vi "Drift_from_ims.vi"(4 "Filename_2":path, 5 "Python Directory Path":path=path "", 6 "Image Channel":string, 7 "Filename_1":path) -> (0 "Error":sgl, 1 "Shift_z (m/s)":sgl, 2 "Shift_x (m/s)":sgl, 3 "Shift_y (m/s)":sgl)   [LabVIEW 2025]
panel:
  out "result string":string
  out "Shift_z (m)":sgl
  out "standard error":string
  out "Shift_x (m)":sgl
  out "Shift_y (m)":sgl
  out "Time Between Scans":sgl
  out "standard output":string
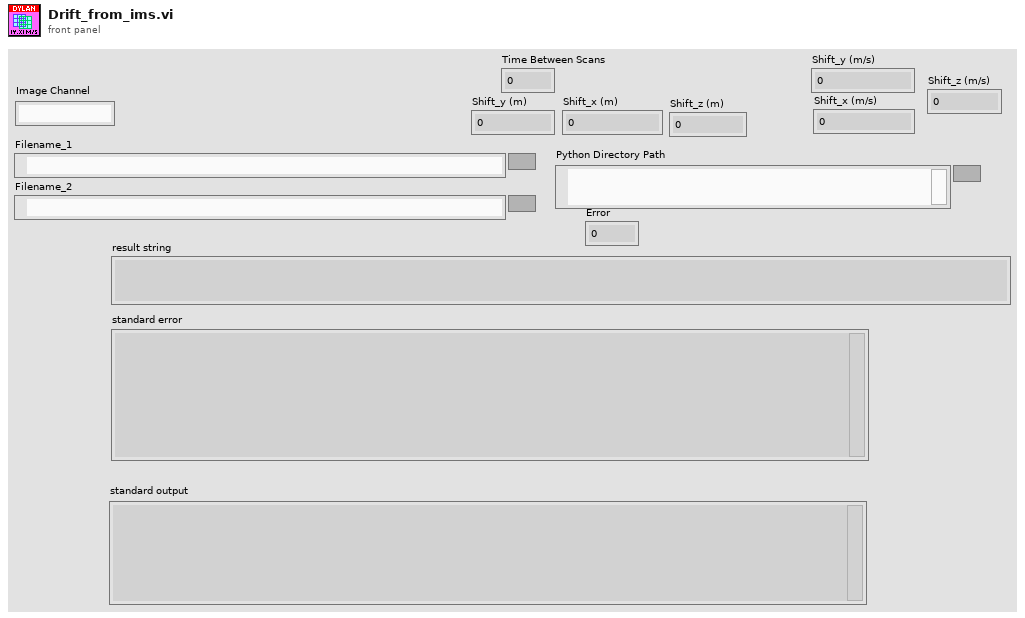
[diagram p1: front panel]
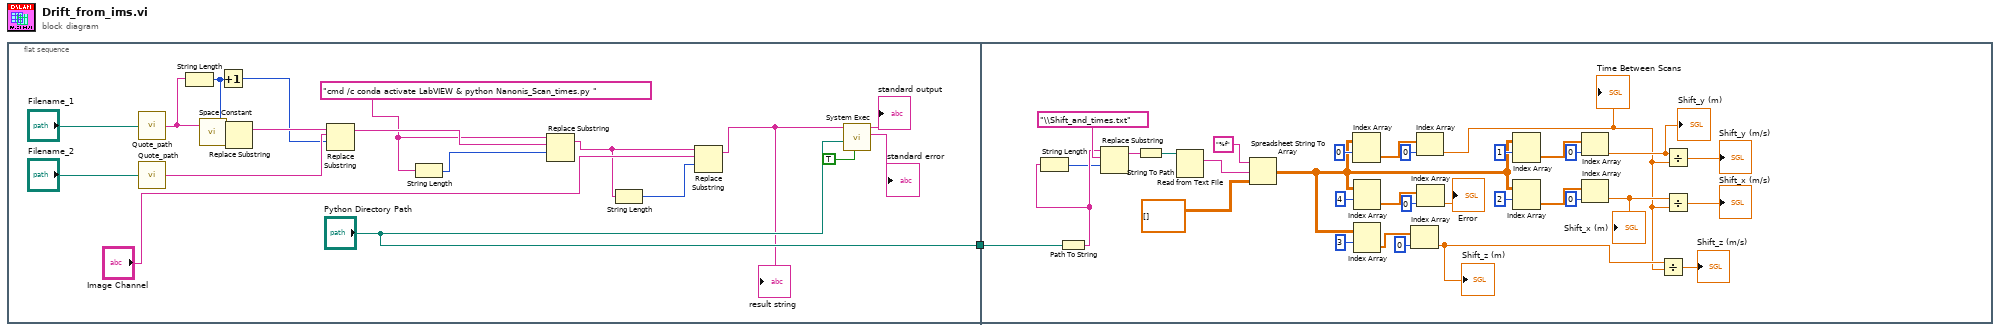
[diagram p0: block diagram]
diagram:
  n1 = flat-sequence {
    tunnel: ["Python Directory Path"] -> w1
    tunnel: w1 -> [w33]
    frame #0 {
      w8 = "cmd /c conda activate LabVIEW & python Nanonis_Scan_times.py " ("command line")
      n2 = call "Quote_path.vi"("File path in"="Filename_1") -> ("result string"=w19:string)
      n3 = call "Quote_path.vi"("File path in"="Filename_2") -> ("result string"=w20:string)
      n4 = String Length(string=w19) -> (length=w17:i32)
      n5 = call <vilib>:"Space Constant.vi"() -> ("String"=w18:string)
      n6 = Increment(x=w17) -> (x+1=w15:i32)
      n7 = Replace Substring(3:w17, 4:w18, 5:w19) -> (1:w16:string)  [unwired: 1 in, 1 out]
      n8 = Replace Substring(3:w15, 4:w20, 5:w16) -> (1:w14:string)  [unwired: 1 in, 1 out]
      n9 = String Length(string=w8) -> (length=w13:i32)
      n10 = Replace Substring(3:w13, 4:w14, 5:w8) -> (1:w4:string)  [unwired: 1 in, 1 out]
      n11 = String Length(string=w4) -> (length=w3:i32)
      n12 = Replace Substring(3:w3, 4:"Image Channel", 5:w4) -> (1:w2:string)  [unwired: 1 in, 1 out]
      "result string" <- w2
      n13 = call <vilib>:"System Exec.vi"("run minimized? (F)"=TRUE, "working directory"="Python Directory Path", "command line"=w2) -> ("standard error"=→"standard error":string, "standard output"=→"standard output":string)  [unwired: 5 in, 2 out]
    }
    frame #1 {
      n14 = Path To String(path=w33) -> (string=w30:string)
      n15 = String Length(string=w30) -> (length=w29:i32)
      n16 = Replace Substring(3:w29, 4:"\\Shift_and_times.txt" ("substring (\"\")"), 5:w30) -> (1:w32:string)  [unwired: 1 in, 1 out]
      n17 = String To Path(string=w32) -> (path=w53:path)
      n18 = Read from Text File(file (use dialog)=w53) -> (text=w52:string)  [unwired: 3 in, 3 out]
      n19 = Spreadsheet String To Array(format string="%f", spreadsheet string=w52, array type (2D Dbl)=sgl[][] []) -> (array=w27:sgl[][])  [unwired: 1 in]
      n20 = Index Array(array=w27, index (row)=0) -> (element=w46:sgl[])  [unwired: 1 in]
      n21 = Index Array(array=w27, index (row)=4) -> (element=w43:sgl[])  [unwired: 1 in]
      n22 = Index Array(array=w27, index (row)=3) -> (element=w24:sgl[])  [unwired: 1 in]
      n23 = Index Array(array=w24, index=0) -> (element=w23:sgl)
      "Shift_z (m)" <- w23
      n24 = Index Array(array=w46, index=0) -> (element=w22:sgl)
      "Time Between Scans" <- w22
      n25 = Index Array(array=w43, index=0) -> (element=→"Error":sgl)
      n26 = Index Array(array=w27, index (row)=1) -> (element=w41:sgl[])  [unwired: 1 in]
      n27 = Index Array(array=w27, index (row)=2) -> (element=w39:sgl[])  [unwired: 1 in]
      n28 = Index Array(array=w41, index=0) -> (element=w34:sgl)
      "Shift_y (m)" <- w34
      n29 = Index Array(array=w39, index=0) -> (element=w37:sgl)
      "Shift_x (m)" <- w37
      n30 = Divide(x=w23, y=w22) -> (x/y=→"Shift_z (m/s)":sgl)
      n31 = Divide(x=w34, y=w22) -> (x/y=→"Shift_y (m/s)":sgl)
      n32 = Divide(x=w37, y=w22) -> (x/y=→"Shift_x (m/s)":sgl)
    }
  }
